vi "rydh-test1.vi"() -> ()   [LabVIEW 2018]
uses:
  Users/Nanocal/Desktop/Calorimetry v1.3/MCL.lvlibp
  Users/Nanocal/Desktop/Calorimetry v1.3/MCL.lvlibp/SynkTek FPGA/FPGA_SharedResources/FPGASharedResources_Lockin_Typedef.ctl
  Users/Nanocal/Desktop/Calorimetry v1.3/MCL.lvlibp/SynkTek FPGA/FPGA_SharedResources/FPGA_SharedResources.lvlib
  Users/Nanocal/Desktop/Calorimetry v1.3/MCL.lvlibp/SynkTek FPGA/FPGA_SharedResources/FPGASharedResources_FreqCtrl_FreqGenTypedef.ctl
  Users/Nanocal/Desktop/Calorimetry v1.3/MCL.lvlibp/SynkTek FPGA/FPGA_SharedResources/FPGASharedResources_CompositeFrequency.ctl
  Users/Nanocal/Desktop/Calorimetry v1.3/MCL.lvlibp/SynkTek Host/LIControl/LIControl_LockinTimeConstant_typedef.ctl
  Users/Nanocal/Desktop/Calorimetry v1.3/MCL.lvlibp/SynkTek Host/LIControl/LIControl.lvlib
  Users/Nanocal/Desktop/Calorimetry v1.3/MCL.lvlibp/SynkTek FPGA/FPGA_SharedResources/FPGASharedResources_HarmonicTypdef.ctl
  Users/Nanocal/Desktop/Calorimetry v1.3/MCL.lvlibp/SynkTek FPGA/FPGA_SharedResources/FPGASharedResources_LockinTypeTypedef.ctl
  Users/Nanocal/Desktop/Calorimetry v1.3/MCL.lvlibp/SynkTek FPGA/FPGA_SharedResources/FPGASharedResources_PhaseShiftCtrl_Typedef.ctl
  Users/Nanocal/Desktop/Calorimetry v1.3/MCL.lvlibp/SynkTek FPGA/FPGA_SharedResources/FPGASharedResources_DutyCycleCtrl_Typedef.ctl
  Users/Nanocal/Desktop/Calorimetry v1.3/MCL.lvlibp/SynkTek Host/LIControl/LIControl_LockinCtrl_typedef.ctl
  Users/Nanocal/Desktop/Calorimetry v1.3/MCL.lvlibp/SynkTek Host/LIdata/LIData_DataReadings_typedef.ctl
  Users/Nanocal/Desktop/Calorimetry v1.3/MCL.lvlibp/SynkTek Host/LIdata/LIData.lvlib
  Users/Nanocal/Desktop/Calorimetry v1.3/MCL.lvlibp/MCL library/MCL_DataRef.ctl
panel:
  in  "MCL object":T1
  out "DataReadings":T2 {"theta (deg)" format="%_7g"; "R" format="%_7g"; "Y" format="%_7g"; "X" format="%_7g"; "DC" format="%_7g"}
  in  "LockinCtrl":T3={"Frequency generator"=enum."Frequency 8", "Time constant (s)"=1.0, "Exponential low-pass filter"={"Enabled"=TRUE, "Stage 1 time const. (s)"=1.0, "Stage 2 time const. (s)"=3.0}, "Harmonic"=1, "Type"=enum."Sine", "Phase shift"=enum."Phase 1", "Duty cycle"=enum."DutyCycle 1"} {"Exponential low-pass filter"."Stage 2 time const. (s)" items=["100 s"=100.0, "50 s"=50.0, "20 s"=20.0, "10 s"=10.0, "5 s"=5.0, "3 s"=3.0, "2 s"=2.0, "1 s"=1.0, "0.5 s"=0.5, "0.3 s"=0.3, "0.2 s"=0.2, "0.1 s"=0.1, "50 ms"=0.05, "20 ms"=0.02, "10 ms"=0.01, "5 ms"=0.005, "2 ms"=0.002, "1 ms"=0.001]; "Exponential low-pass filter"."Stage 1 time const. (s)" items=["100 s"=100.0, "50 s"=50.0, "20 s"=20.0, "10 s"=10.0, "5 s"=5.0, "3 s"=3.0, "2 s"=2.0, "1 s"=1.0, "0.5 s"=0.5, "0.3 s"=0.3, "0.2 s"=0.2, "0.1 s"=0.1, "50 ms"=0.05, "20 ms"=0.02, "10 ms"=0.01, "5 ms"=0.005, "2 ms"=0.002, "1 ms"=0.001]; "Time constant (s)" items=["100 s"=100.0, "50 s"=50.0, "20 s"=20.0, "10 s"=10.0, "5 s"=5.0, "3 s"=3.0, "2 s"=2.0, "1 s"=1.0, "0.5 s"=0.5, "0.3 s"=0.3, "0.2 s"=0.2, "0.1 s"=0.1, "50 ms"=0.05, "20 ms"=0.02, "10 ms"=0.01, "5 ms"=0.005, "2 ms"=0.002, "1 ms"=0.001]}
  in  "Composite frequency":T10
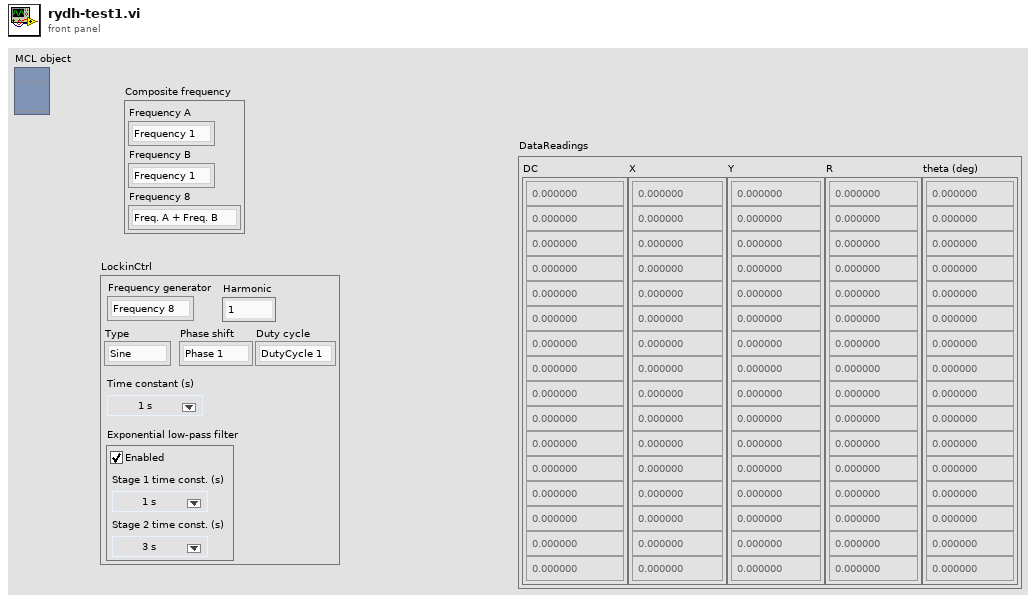
[diagram p1: front panel]
types:
  T1 = typedef "MCL.lvlibp/MCL_DataRef.ctl" = refnum<vi>
  T2 = typedef "MCL.lvlibp/LIData.lvlib/LIData_DataReadings_typedef.ctl" = cluster{"DC":dbl[], "X":dbl[], "Y":dbl[], "R":dbl[], "theta (deg)":dbl[]}
  T3 = typedef "MCL.lvlibp/LIControl.lvlib/LIControl_LockinCtrl_typedef.ctl" = cluster{"Frequency generator":T4, "Time constant (s)":T5, "Exponential low-pass filter":cluster{"Enabled":bool, "Stage 1 time const. (s)":T5, "Stage 2 time const. (s)":T5}, "Harmonic":T6, "Type":T7, "Phase shift":T8, "Duty cycle":T9}
  T4 = typedef "MCL.lvlibp/FPGA_SharedResources.lvlib/FPGASharedResources_FreqCtrl_FreqGenTypedef.ctl" = enum8{"Frequency 1", "Frequency 2", "Frequency 3", "Frequency 4", "Frequency 5", "Frequency 6: PLL 1", "Frequency 7: PLL 2", "Frequency 8"}
  T5 = typedef "MCL.lvlibp/LIControl.lvlib/LIControl_LockinTimeConstant_typedef.ctl" = dbl
  T6 = typedef "MCL.lvlibp/FPGA_SharedResources.lvlib/FPGASharedResources_HarmonicTypdef.ctl" = u16
  T7 = typedef "MCL.lvlibp/FPGA_SharedResources.lvlib/FPGASharedResources_LockinTypeTypedef.ctl" = enum8{"Sine", "Square", "Boxcar"}
  T8 = typedef "MCL.lvlibp/FPGA_SharedResources.lvlib/FPGASharedResources_PhaseShiftCtrl_Typedef.ctl" = enum8{"Phase 1", "Phase 2", "Phase 3", "Phase 4", "Phase 5", "Phase 6", "Phase 7", "Disabled"}
  T9 = typedef "MCL.lvlibp/FPGA_SharedResources.lvlib/FPGASharedResources_DutyCycleCtrl_Typedef.ctl" = enum8{"DutyCycle 1", "DutyCycle 2", "DutyCycle 3", "DutyCycle 4", "DutyCycle 5", "DutyCycle 6", "DutyCycle 7", "Inactive"}
  T10 = typedef "MCL.lvlibp/FPGA_SharedResources.lvlib/FPGASharedResources_CompositeFrequency.ctl" = cluster{"Frequency A":T4, "Frequency B":T4, "Frequency 8":enum8{"Freq. A + Freq. B", "Freq. A - Freq. B"}}
  T11 = typedef "MCL.lvlibp/FPGA_SharedResources.lvlib/FPGASharedResources_Lockin_Typedef.ctl" = enum8{"Lock-in set L1", "Lock-in set L2"}
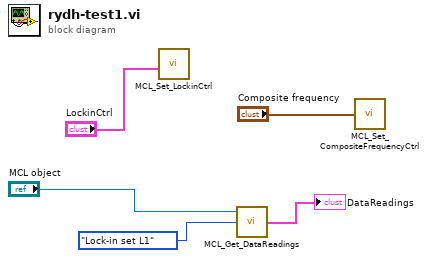
[diagram p0: block diagram]
diagram:
  n1 = call "MCL_Set_LockinCtrl.vi"("LockinCtrl"="LockinCtrl") -> ()  [unwired: 5 in, 2 out]
  n2 = call "MCL_Get_DataReadings.vi"("Lockin"=FPGASharedResources_Lockin_Typedef."Lock-in set L1", "MCL object"="MCL object") -> ("DataReadings"=→"DataReadings":T2)  [unwired: 1 in, 2 out]
  n3 = call "MCL_Set_CompositeFrequencyCtrl.vi"("Composite frequency"="Composite frequency") -> ()  [unwired: 3 in, 2 out]
